vi "Append Device to List.vi"(8 "Error In":errorcluster, 10 "Device":refnum<class "Device.lvclass">, 11 "Device List State":T1) -> (0 "Error Out":errorcluster, 3 "Device List State out":T1)   [LabVIEW 2015]
uses:
  Device/Device.lvclass
  Device List State.ctl
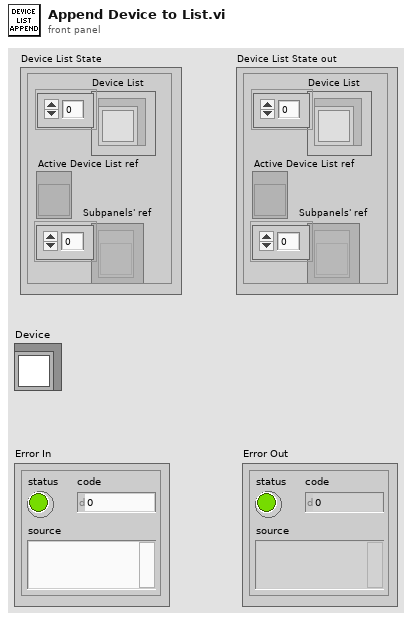
[diagram p1: front panel]
types:
  T1 = typedef "Device List State.ctl" = cluster{"Device List":refnum<class "Device.lvclass">[], "Active Device List ref":refnum<vi>, "Subpanels' ref":refnum<vi>[]}
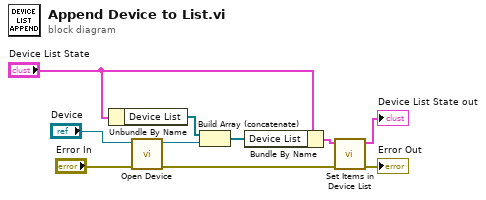
[diagram p0: block diagram]
diagram:
  n1 = Unbundle By Name("Device List State") -> ("Device List"=w7:refnum<class "Device.lvclass">[])
  n2 = call "Open Device.vi"("error in (no error)"="Error In", "Device"="Device") -> ("error out"=w3:errorcluster, "Device out"=w8:refnum<class "Device.lvclass">)  [unwired: 8 in]
  n3 = Build Array (concatenate)(w7, w8) -> (w5:refnum<class "Device.lvclass">[])
  n4 = Bundle By Name(cluster="Device List State", "Device List"=w5) -> (w4:T1)
  n5 = call "Set Items in Device List.vi"("Error In"=w3, "Device List State"=w4) -> ("Error Out"=→"Error Out":errorcluster, "Device List State out"=→"Device List State out":T1)  [unwired: 8 in]
